vi "Analysis.vi"(8 "error in":errorcluster, 10 "IN":T1) -> (0 "error out":errorcluster, 3 "OUT":cluster{"FWHMx (um)":dbl, "FWHMy (um)":dbl})   [LabVIEW 2020]
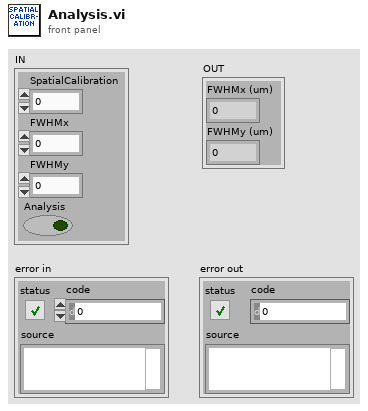
[diagram p1: front panel]
types:
  T1 = cluster{"SpatialCalibration":dbl, "FWHMx":dbl, "FWHMy":dbl, "Analysis":bool}
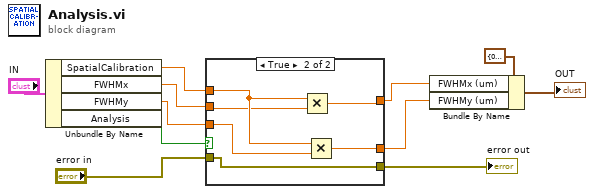
[diagram p0: block diagram]
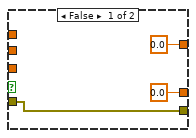
[diagram p2: hidden frame]
diagram:
  n1 = Unbundle By Name("IN") -> ("SpatialCalibration"=w5:dbl, "FWHMx"=w4:dbl, "FWHMy"=w3:dbl, "Analysis"=w1:bool)
  n2 = case shown="True" w1 {
    tunnel: w5 -> [_ w20]
    tunnel: w4 -> [_ w19]
    tunnel: w3 -> [_ w18]
    tunnel: [0.0 w17] -> w8
    tunnel: [0.0 w16] -> w7
    tunnel: "error in" -> [w12 w15]
    tunnel: [w12 w15] -> w11
    frame False {
    }
    frame True {
      n3 = Multiply(x=w20, y=w19) -> (x*y=w17:dbl)
      n4 = Multiply(x=w20, y=w18) -> (x*y=w16:dbl)
    }
  }
  "error out" <- w11
  n5 = Bundle By Name(cluster=cluster{"FWHMx (um)":dbl, "FWHMy (um)":dbl} {"FWHMx (um)"=0.0, "FWHMy (um)"=0.0} ("OUT"), "FWHMx (um)"=w8, "FWHMy (um)"=w7) -> (→"OUT":cluster{"FWHMx (um)":dbl, "FWHMy (um)":dbl})
